vi "vizu_XY2.vi"() -> ()   [LabVIEW 2013]
uses:
  <vilib>/Analysis/Matrix/Datatypes/RealMatrix.ctl
  <vilib>/Analysis/Matrix/Numeric/Conversions/Matrix To Array - RM.vi
  <vilib>/Analysis/Matrix/NI_Matrix.lvlib
panel:
  in  "LY":dbl
  in  "LX":dbl format="%#_13g"
  out "Graphe XY":T1(graph)
  in  "stored XY":T2
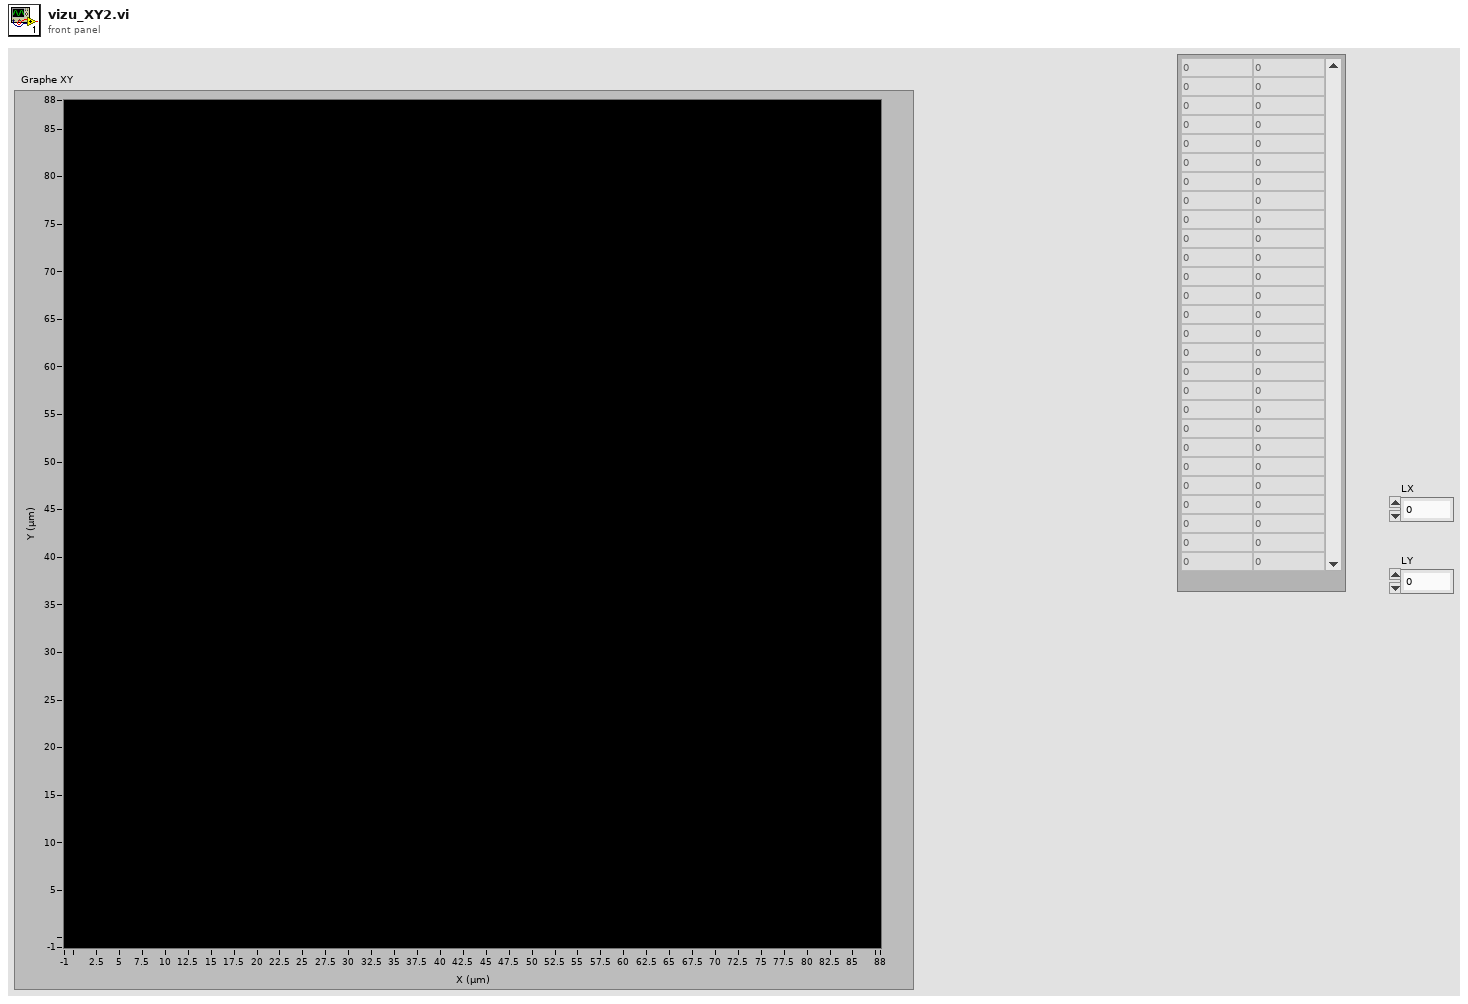
[diagram p1: front panel]
types:
  T1 = cluster{cluster{"Real Matrix Element":dbl, dbl}[]}[]
  T2 = typedef "NI_Matrix.lvlib/RealMatrix.ctl" = dbl[][]
  T3 = cluster{"Real Matrix Element":dbl, "Real Matrix Element":dbl}
  T4 = cluster{cluster{"Real Matrix Element":dbl, "Real Matrix Element":dbl}[]}
  T5 = cluster{cluster{"Real Matrix Element":dbl, "Real Matrix Element":dbl}[]}[]
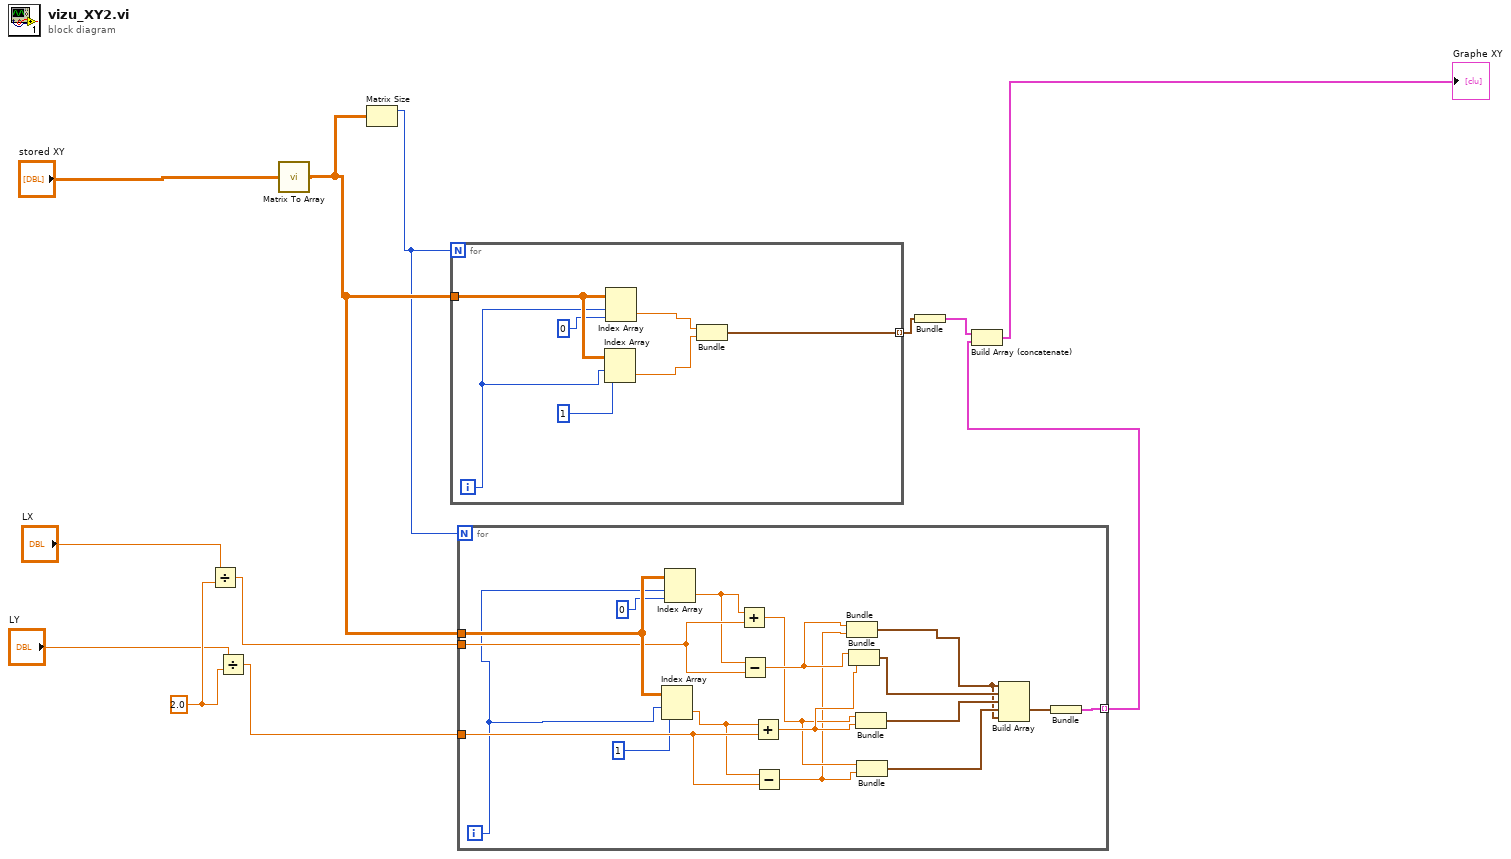
[diagram p0: block diagram]
diagram:
  w8 = 2.0
  n1 = Divide(x="LX", y=w8) -> (x/y=w7:dbl)
  n2 = Divide(x="LY", y=w8) -> (x/y=w6:dbl)
  n3 = call-poly <vilib>:"Matrix To Array.vi"("Real Matrix"="stored XY") -> ("Real 2D Array"=w9:dbl[][])
  n4 = Matrix Size(0:w9) -> (1:w4:i32)  [unwired: 1 out]
  n5 = for {
    N: w4 -> [_]
    tunnel: w9 -> [w19]
    tunnel: [w15] -> w11 mode=indexing
    i -> [w17]
    n6 = Index Array(array=w19, index (row)=w17, index (col)=1) -> (element=w13:dbl)
    n7 = Index Array(array=w19, index (row)=w17, index (col)=0) -> (element=w14:dbl)
    n8 = Bundle("Real Matrix Element"=w14, "Real Matrix Element"=w13) -> (w15:T3)  [unwired: 1 in]
  }
  n9 = for {
    N: w4 -> [_]
    tunnel: w9 -> [w37]
    tunnel: w7 -> [w36]
    tunnel: w6 -> [w35]
    tunnel: [w34] -> w3 mode=indexing
    i -> [w20]
    n10 = Index Array(array=w37, index (row)=w20, index (col)=1) -> (element=w30:dbl)
    n11 = Index Array(array=w37, index (row)=w20, index (col)=0) -> (element=w31:dbl)
    n12 = Add(x=w31, y=w36) -> (x+y=w27:dbl)
    n13 = Subtract(x=w31, y=w36) -> (x-y=w29:dbl)
    n14 = Add(x=w30, y=w35) -> (x+y=w28:dbl)
    n15 = Subtract(x=w30, y=w35) -> (x-y=w26:dbl)
    n16 = Bundle(w29, w26) -> (w21:cluster{dbl, dbl})  [unwired: 1 in]
    n17 = Bundle(w29, w28) -> (w25:cluster{dbl, dbl})  [unwired: 1 in]
    n18 = Bundle(w27, w28) -> (w24:cluster{dbl, dbl})  [unwired: 1 in]
    n19 = Bundle(w27, w26) -> (w23:cluster{dbl, dbl})  [unwired: 1 in]
    n20 = Build Array(w21, w25, w24, w23, w21) -> (w22:cluster{dbl, dbl}[])
    n21 = Bundle(w22) -> (w34:cluster{cluster{dbl, dbl}[]})  [unwired: 1 in]
  }
  n22 = Bundle(w11) -> (w10:T4)  [unwired: 1 in]
  n23 = Build Array (concatenate)(w10, w3) -> (→"Graphe XY":T5)
